vi "SetItemJustify.vi"(5 "列データ表示位置":enum16{"Left", "Center", "Right"}[](array[ring]), 7 "列オフセット":i32, 8 "error in (no error)":errorcluster caption="エラー入力（エラーなし）", 9 "行数":i32=1, 11 "Table入力":refnum<vi>) -> (0 "error out":errorcluster caption="エラー出力", 3 "Table入力(copy)":refnum<vi>)   [LabVIEW 2014]
uses:
  <vilib>/Utility/miscctls.llb/LVRowAndColumnTypeDef.ctl
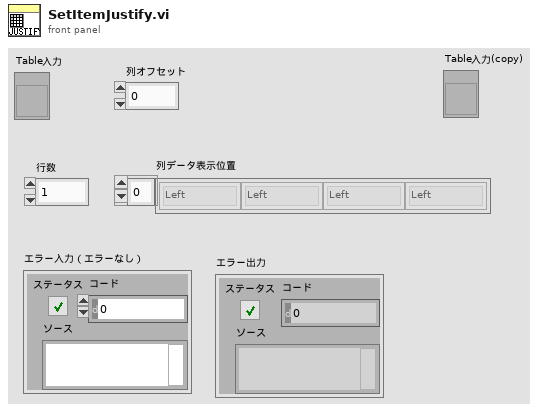
[diagram p1: front panel]
types:
  T1 = typedef "LVRowAndColumnTypeDef.ctl" = cluster{"Row":i32, "Column":i32}
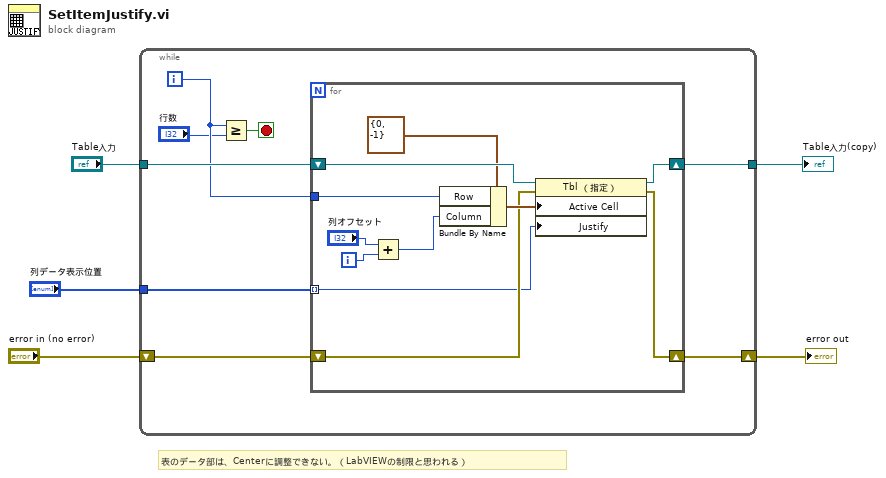
[diagram p0: block diagram]
diagram:
  # "表のデータ部は、Centerに調整できない。（LabVIEWの制限と思われる）"
  n1 = while {
    tunnel: "列データ表示位置" -> [w13]
    tunnel: "Table入力" -> [w12]
    tunnel: [w10] -> w3
    shift-right: [w8] -> w1
    shift-left: "error in (no error)" -> [w9]
    i -> [w7]
    stop <- w11 stop-if-true
    n2 = Greater Or Equal?(x=w7, y="行数") -> (x >= y?=w11:bool)
    n3 = for {
      tunnel: w13 -> [w14] mode=indexing
      tunnel: w7 -> [w18]
      shift-right: [w17] -> w10
      shift-left: w12 -> [w24]
      shift-right: [w15] -> w8
      shift-left: w9 -> [w16]
      i -> [w20]
      n4 = Add(x="列オフセット", y=w20) -> (x+y=w19:i32)
      n5 = Bundle By Name(cluster=T1 {"Row"=0, "Column"=-1} ("アクティブセル:アクティブセル"), "Row"=w18, "Column"=w19) -> (w22:T1)
      n6 = property class="Tbl （指定）"(reference=w24, error in=w16, "Active Cell"=w22, "Justify"=w14) -> (reference out=w17:refnum<vi>, error out=w15:errorcluster)
    }
  }
  "Table入力(copy)" <- w3
  "error out" <- w1
